vi "FR Do Single Measurement.vi"(6 "Iteration index":i32, 7 "TWM handle in":i32, 8 "error in (no error)":errorcluster, 11 "FFmeter settings in":T1 {"Measurement properties"."Record length (multiples of period)" format="%#_3p"; "Measurement properties"."Sampling frequency (Hz)" format="%#_3p"; "Measurement properties"."Measurement frequencies (Hz)" format="%#_3p"}) -> (0 "error out":errorcluster, 1 "TWM result as string":string[][](array[string]), 2 "DC readings":dbl[](array[numeric]), 3 "FFmeter settings out":T1 {"Measurement properties"."Record length (multiples of period)" format="%#_3p"; "Measurement properties"."Sampling frequency (Hz)" format="%#_3p"; "Measurement properties"."Measurement frequencies (Hz)" format="%#_3p"}, 5 "TWM handle out":i32)   [LabVIEW 2020]
doc: "Makes a single measurement in TWM and multimeter DC readings. Either in parallel, or in series."
uses:
  FR GUI/Type definitions/FFmeter settings.ctl
  General AC source/Type definitions/AC Source.ctl
  General AC source/Type definitions/AC Source type.ctl
  General DC meter/Type definitions/DC meter.ctl
  General DC meter/Type definitions/DC meter type.ctl
  Type definitions/FR Measuement properties.ctl
  FR Utilities/Type definitions/FR Template definition.ctl
  Utilities/Type definitions/Sampling properties.ctl
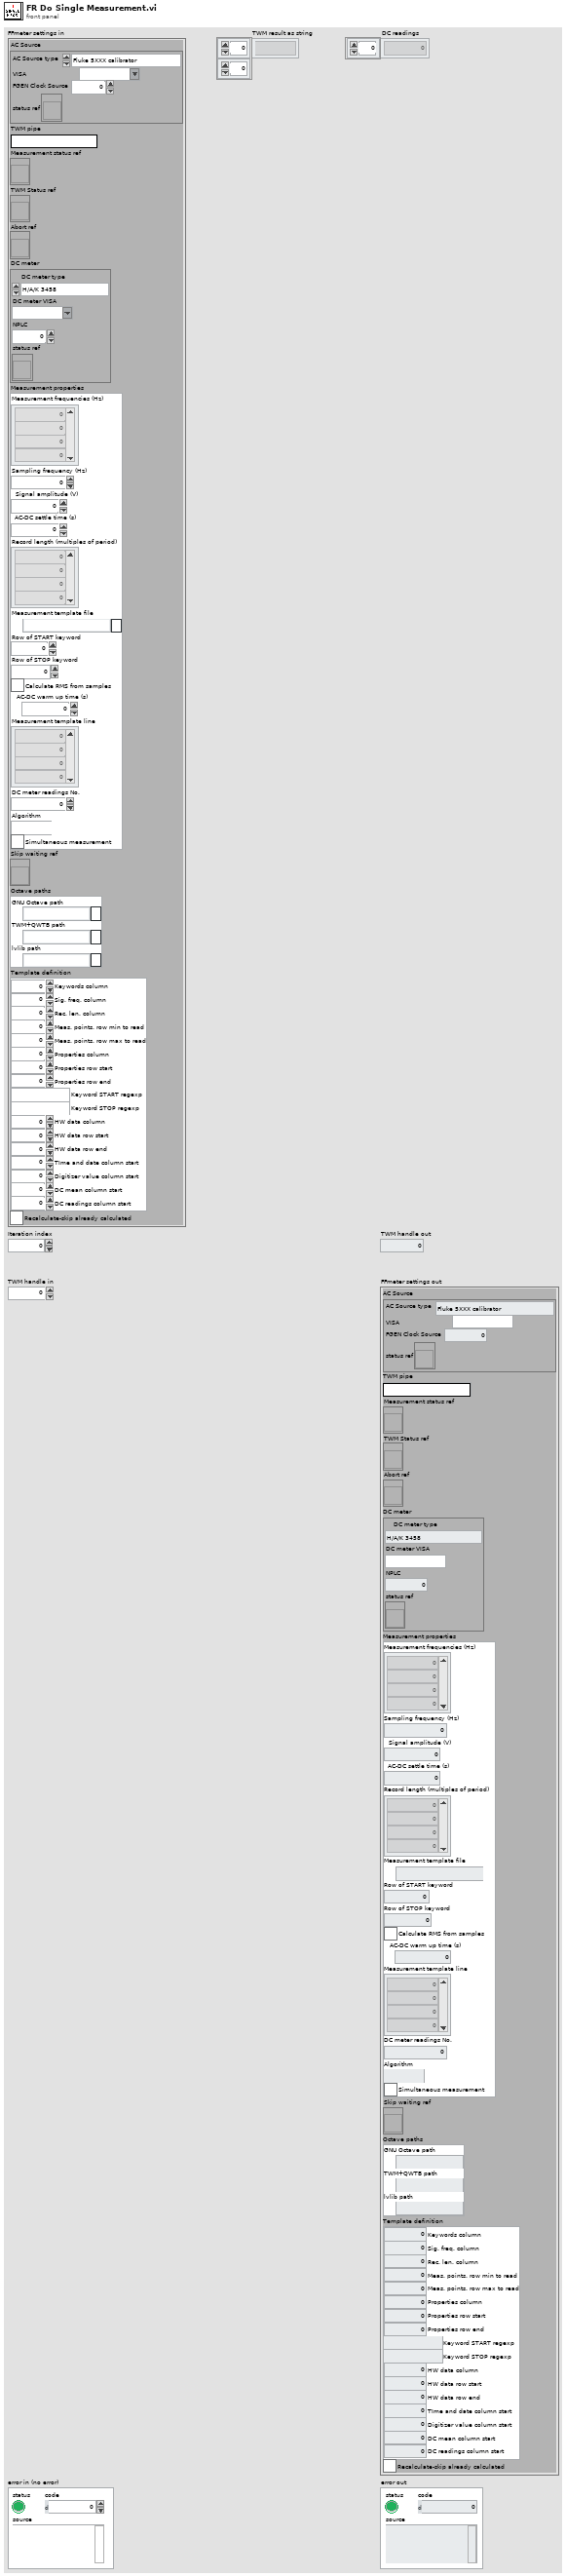
[diagram p1: front panel]
types:
  T1 = typedef "FFmeter settings.ctl" = cluster{"AC Source":T2, "TWM pipe":string, "Measurement status ref":refnum<vi>, "TWM Status ref":refnum<vi>, "Abort ref":refnum<vi>, "DC meter":T4, "Measurement properties":T6, "Skip waiting ref":refnum<vi>, "Octave paths":cluster{"GNU Octave path":path, "TWM+QWTB path":path, "lvlib path":path}, "Template definition":T7, "Recalculate-skip already calculated":bool}
  T2 = typedef "AC Source.ctl" = cluster{"AC Source type":T3, "VISA":refnum<visa-resource-name>, "Ref. clock (Hz)":dbl, "status ref":refnum<vi>}
  T3 = typedef "AC Source type.ctl" = enum16{"Fluke 5XXX calibrator", "Tektronix AFG3000 series", "dummy"}
  T4 = typedef "DC meter.ctl" = cluster{"DC meter type":T5, "DC meter VISA":refnum<visa-resource-name>, "NPLC":i32, "status ref":refnum<vi>}
  T5 = typedef "DC meter type.ctl" = enum16{"H/A/K 3458", "Fluke 8508A", "dummy", "Keithley 2182"}
  T6 = typedef "FR Measuement properties.ctl" = cluster{"Measurement frequencies (Hz)":dbl[], "Sampling frequency (Hz)":dbl, "Signal amplitude (V)":dbl, "AC-DC settle time (s)":dbl, "Record length (multiples of period)":dbl[], "Measurement template file":path, "Row of START keyword":i32, "Row of STOP keyword":i32, "Calculate RMS from samples":bool, "AC-DC warm up time (s)":dbl, "Measurement template line":i32[], "DC meter readings No.":i32, "Algorithm":string, "Simultaneous measurement":bool}
  T7 = typedef "FR Template definition.ctl" = cluster{"Keywords column":i32, "Sig. freq. column":i32, "Rec. len. column":i32, "Meas. points. row min to read":i32, "Meas. points. row max to read":i32, "Properties column":i32, "Properties row start":i32, "Properties row end":i32, "Keyword START regexp":string, "Keyword STOP regexp":string, "HW data column":i32, "HW data row start":i32, "HW data row end":i32, "TIme and date column start":i32, "Digitizer value column start ":i32, "DC mean column start ":i32, "DC readings column start":i32}
  T8 = typedef "Sampling properties.ctl" = cluster{"Sampling frequency (Hz)":dbl, "Record length (multiples of period)":dbl, "Signal amplitude (V)":dbl, "Measurement frequency (Hz)":dbl, "Calculate RMS from samples":bool, "Algorithm":string, "Measurement path":string}
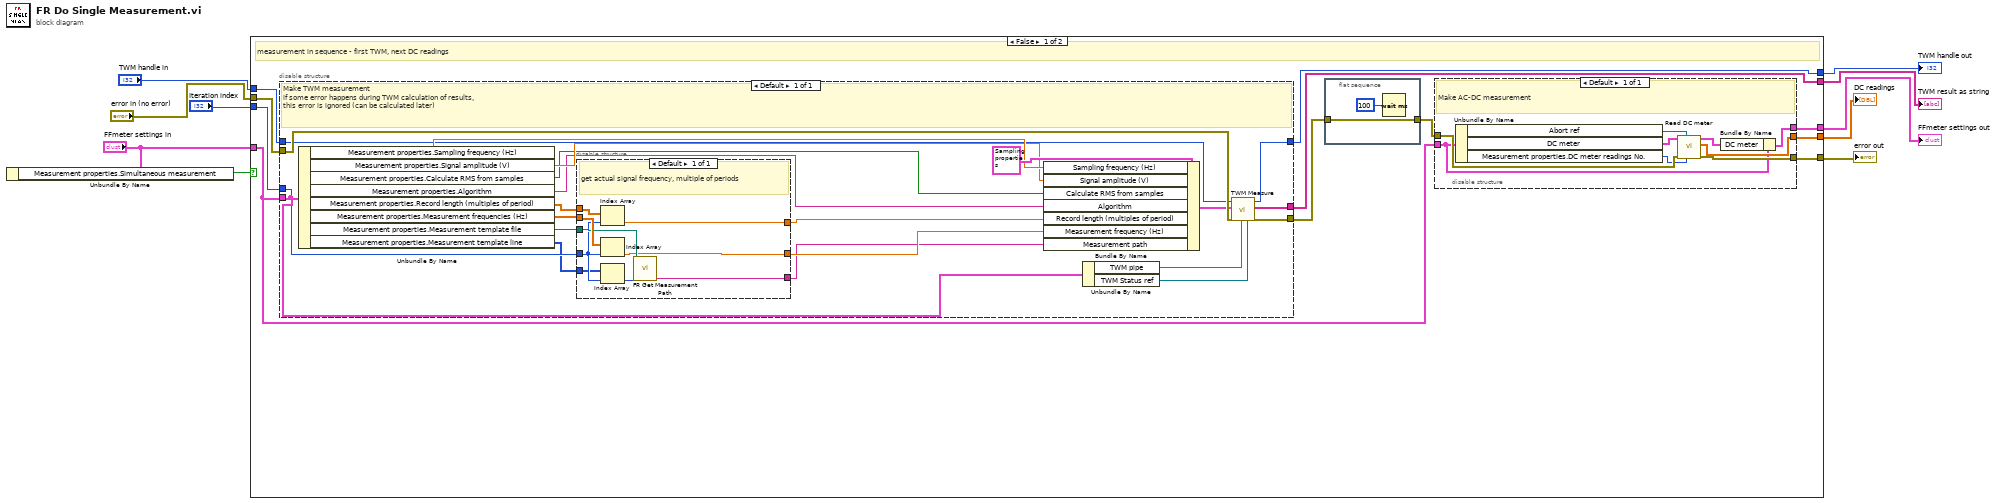
[diagram p0: block diagram]
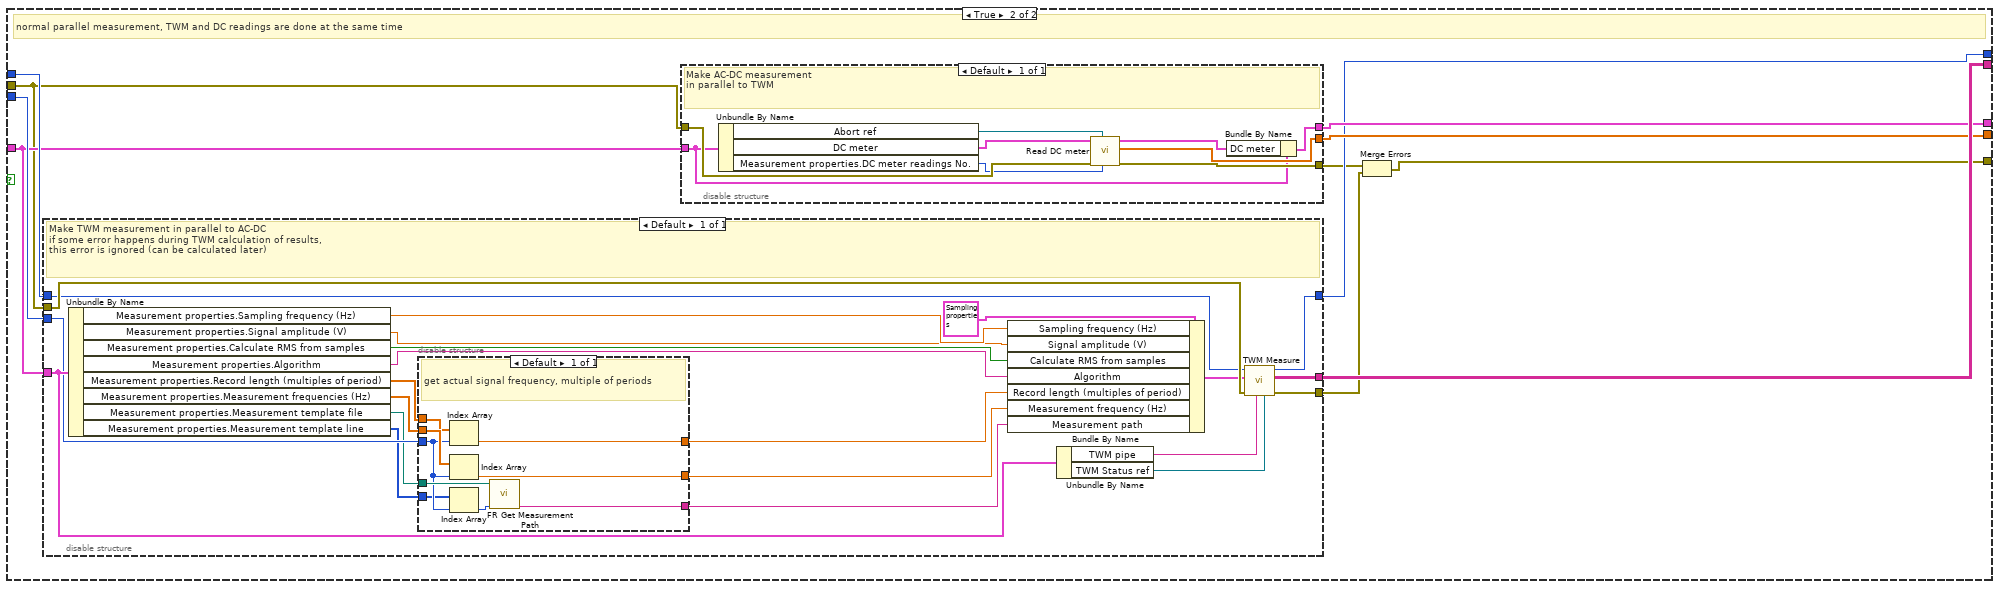
[diagram p2: hidden frame]
diagram:
  n1 = Unbundle By Name("FFmeter settings in") -> ("Measurement properties.Simultaneous measurement"=w1:bool)
  n2 = case shown="False" w1 {
    tunnel: "Iteration index" -> [w20 w74]
    tunnel: "TWM handle in" -> [w21 w73]
    tunnel: [w15 w72] -> w8
    tunnel: [w18 w71] -> w7
    tunnel: [w17 w70] -> w6
    tunnel: [w16 w69] -> w5
    tunnel: "FFmeter settings in" -> [w14 w68]
    tunnel: "error in (no error)" -> [w19 w67]
    tunnel: [w13 w64] -> w3
    frame False {
      # "measurement in sequence - first TWM, next DC readings"
      n3 = disable-structure shown="Default" {
        disable-tunnel: [w52] -> w11
        disable-tunnel: w19 -> [w54]
        disable-tunnel: w14 -> [w46]
        disable-tunnel: w21 -> [w33]
        disable-tunnel: [w51] -> w16
        disable-tunnel: w20 -> [w45]
        disable-tunnel: [w53] -> w15
        frame Enabled {
          # "Make TWM measurement\nif some error happens during TWM calculation of results,\nthis error is ignored (can be calculated later)"
          n4 = Unbundle By Name(w46) -> ("Measurement properties.Sampling frequency (Hz)"=w44:dbl, "Measurement properties.Signal amplitude (V)"=w38:dbl, "Measurement properties.Calculate RMS from samples"=w37:bool, "Measurement properties.Algorithm"=w36:string, "Measurement properties.Record length (multiples of period)"=w43:dbl[], "Measurement properties.Measurement frequencies (Hz)"=w42:dbl[], "Measurement properties.Measurement template file"=w35:path, "Measurement properties.Measurement template line"=w34:i32[])
          n5 = disable-structure shown="Default" {
            disable-tunnel: w42 -> [w63]
            disable-tunnel: w43 -> [w62]
            disable-tunnel: w45 -> [w59]
            disable-tunnel: [w61] -> w39
            disable-tunnel: w35 -> [w60]
            disable-tunnel: w34 -> [w58]
            disable-tunnel: [w56] -> w41
            disable-tunnel: [w55] -> w40
            frame Enabled {
              # "get actual signal frequency, multiple of periods"
              n6 = Index Array(array=w62, index=w59) -> (element=w55:dbl)
              n7 = Index Array(array=w63, index=w59) -> (element=w56:dbl)
              n8 = Index Array(array=w58, index=w59) -> (element=w57:i32)
              n9 = call "FR Get Measurement Path.vi"("Template line"=w57, "Measurement template file"=w60) -> ("Measurement path as string"=w61:string)  [unwired: 8 in, 1 out]
            }
          }
          n10 = Bundle By Name(cluster=T8 {"Sampling frequency (Hz)"=500000.0, "Record length (multiples of period)"=1000.0, "Signal amplitude (V)"=4.5, "Measurement frequency (Hz)"=1000.0, "Calculate RMS from samples"=FALSE, "Algorithm"="TWM-WFFT", "Measurement path"=""} ("TWM Measurement properties"), "Sampling frequency (Hz)"=w44, "Signal amplitude (V)"=w38, "Calculate RMS from samples"=w37, "Algorithm"=w36, "Record length (multiples of period)"=w40, "Measurement frequency (Hz)"=w41, "Measurement path"=w39) -> (w47:T8)
          n11 = Unbundle By Name(w46) -> ("TWM pipe"=w50:string, "TWM Status ref"=w49:refnum<vi>)
          n12 = call "TWM Measure.vi"("TWM Status ref"=w49, "TWM pipe"=w50, "error in (no error)"=w54, "TWM Measurement properties"=w47, "TWM handle"=w33) -> ("error out"=w52:errorcluster, "TWM result as string"=w53:string[][], "TWM handle out"=w51:i32)  [unwired: 4 in]
        }
      }
      n13 = flat-sequence {
        tunnel: [w22] -> w12
        tunnel: w11 -> [w22]
        frame #0 {
          n14 = Wait (ms)(milliseconds to wait=u32 100) -> ()  [unwired: 1 out]
        }
      }
      n15 = disable-structure shown="Default" {
        disable-tunnel: [w32] -> w18
        disable-tunnel: [w31] -> w13
        disable-tunnel: w12 -> [w30]
        disable-tunnel: w14 -> [w27]
        disable-tunnel: [w26] -> w17
        frame Enabled {
          # "Make AC-DC measurement"
          n16 = Unbundle By Name(w27) -> ("Abort ref"=w25:refnum<vi>, "DC meter"=w29:T4, "Measurement properties.DC meter readings No."=w24:i32)
          n17 = call "Read DC meter.vi"("No of readings"=w24, "abort reference"=w25, "error in (no error)"=w30, "DC meter"=w29) -> ("error out"=w31:errorcluster, "DC readings"=w32:dbl[], "DC meter out"=w28:T4)  [unwired: 5 in]
          n18 = Bundle By Name(cluster=w27, "DC meter"=w28) -> (w26:T1)
        }
      }
    }
    frame True {
      # "normal parallel measurement, TWM and DC readings are done at the same time"
      n19 = disable-structure shown="Default" {
        disable-tunnel: [w103] -> w65
        disable-tunnel: w67 -> [w105]
        disable-tunnel: w68 -> [w97]
        disable-tunnel: w73 -> [w84]
        disable-tunnel: [w102] -> w69
        disable-tunnel: w74 -> [w96]
        disable-tunnel: [w104] -> w72
        frame Enabled {
          # "Make TWM measurement in parallel to AC-DC\nif some error happens during TWM calculation of results,\nthis error is ignored (can be calculated later)"
          n20 = Unbundle By Name(w97) -> ("Measurement properties.Sampling frequency (Hz)"=w95:dbl, "Measurement properties.Signal amplitude (V)"=w89:dbl, "Measurement properties.Calculate RMS from samples"=w88:bool, "Measurement properties.Algorithm"=w87:string, "Measurement properties.Record length (multiples of period)"=w94:dbl[], "Measurement properties.Measurement frequencies (Hz)"=w93:dbl[], "Measurement properties.Measurement template file"=w86:path, "Measurement properties.Measurement template line"=w85:i32[])
          n21 = disable-structure shown="Default" {
            disable-tunnel: w93 -> [w114]
            disable-tunnel: w94 -> [w113]
            disable-tunnel: w96 -> [w110]
            disable-tunnel: [w112] -> w90
            disable-tunnel: w86 -> [w111]
            disable-tunnel: w85 -> [w109]
            disable-tunnel: [w107] -> w92
            disable-tunnel: [w106] -> w91
            frame Enabled {
              # "get actual signal frequency, multiple of periods"
              n22 = Index Array(array=w113, index=w110) -> (element=w106:dbl)
              n23 = Index Array(array=w114, index=w110) -> (element=w107:dbl)
              n24 = Index Array(array=w109, index=w110) -> (element=w108:i32)
              n25 = call "FR Get Measurement Path.vi"("Template line"=w108, "Measurement template file"=w111) -> ("Measurement path as string"=w112:string)  [unwired: 8 in, 1 out]
            }
          }
          n26 = Bundle By Name(cluster=T8 {"Sampling frequency (Hz)"=500000.0, "Record length (multiples of period)"=1000.0, "Signal amplitude (V)"=4.5, "Measurement frequency (Hz)"=1000.0, "Calculate RMS from samples"=FALSE, "Algorithm"="TWM-WFFT", "Measurement path"=""} ("TWM Measurement properties"), "Sampling frequency (Hz)"=w95, "Signal amplitude (V)"=w89, "Calculate RMS from samples"=w88, "Algorithm"=w87, "Record length (multiples of period)"=w91, "Measurement frequency (Hz)"=w92, "Measurement path"=w90) -> (w98:T8)
          n27 = Unbundle By Name(w97) -> ("TWM pipe"=w101:string, "TWM Status ref"=w100:refnum<vi>)
          n28 = call "TWM Measure.vi"("TWM Status ref"=w100, "TWM pipe"=w101, "error in (no error)"=w105, "TWM Measurement properties"=w98, "TWM handle"=w84) -> ("error out"=w103:errorcluster, "TWM result as string"=w104:string[][], "TWM handle out"=w102:i32)  [unwired: 4 in]
        }
      }
      n29 = disable-structure shown="Default" {
        disable-tunnel: [w83] -> w71
        disable-tunnel: [w82] -> w66
        disable-tunnel: w67 -> [w81]
        disable-tunnel: w68 -> [w78]
        disable-tunnel: [w77] -> w70
        frame Enabled {
          # "Make AC-DC measurement\nin parallel to TWM"
          n30 = Unbundle By Name(w78) -> ("Abort ref"=w76:refnum<vi>, "DC meter"=w80:T4, "Measurement properties.DC meter readings No."=w75:i32)
          n31 = call "Read DC meter.vi"("No of readings"=w75, "abort reference"=w76, "error in (no error)"=w81, "DC meter"=w80) -> ("error out"=w82:errorcluster, "DC readings"=w83:dbl[], "DC meter out"=w79:T4)  [unwired: 5 in]
          n32 = Bundle By Name(cluster=w78, "DC meter"=w79) -> (w77:T1)
        }
      }
      n33 = Merge Errors(w66, w65) -> (w64:errorcluster)
    }
  }
  "TWM result as string" <- w8
  "error out" <- w3
  "DC readings" <- w7
  "FFmeter settings out" <- w6
  "TWM handle out" <- w5
